vi "test4-SyncMessageWithError_API.vi"(8 "error in (no error)":errorcluster, 11 "TestCase in":refnum<class "testcase-CSMMessage.lvclass">) -> (0 "error out":errorcluster, 3 "TestCase out":refnum<class "testcase-CSMMessage.lvclass">)   [LabVIEW 2017, in "testcase-CSMMessage.lvclass"]
uses:
  testcase-CSMMessage.lvclass
  src/user.lib/_NEVSTOP/Communicable State Machine(CSM)/AdvanceAPI/CSM - Make String Arguments Safe.vi
  src/user.lib/_NEVSTOP/Communicable State Machine(CSM)/AdvanceAPI/CSM - Keywords.vi
  <vilib>/addons/_JKI Toolkits/VI Tester/TestCase.llb/TestCase.lvclass
  src/user.lib/_NEVSTOP/Communicable State Machine(CSM)/Communicable State Machine.lvlib
  C:/Program Files (x86)/National Instruments/LabVIEW 2017/vi.lib/addons/_JKI Toolkits/VI Tester/TestCase.llb/TestCase.lvclass
panel:
  out "LoopCount":i32
  out "Source CSM modules":string[](array[string])
  out "concatenated string":string
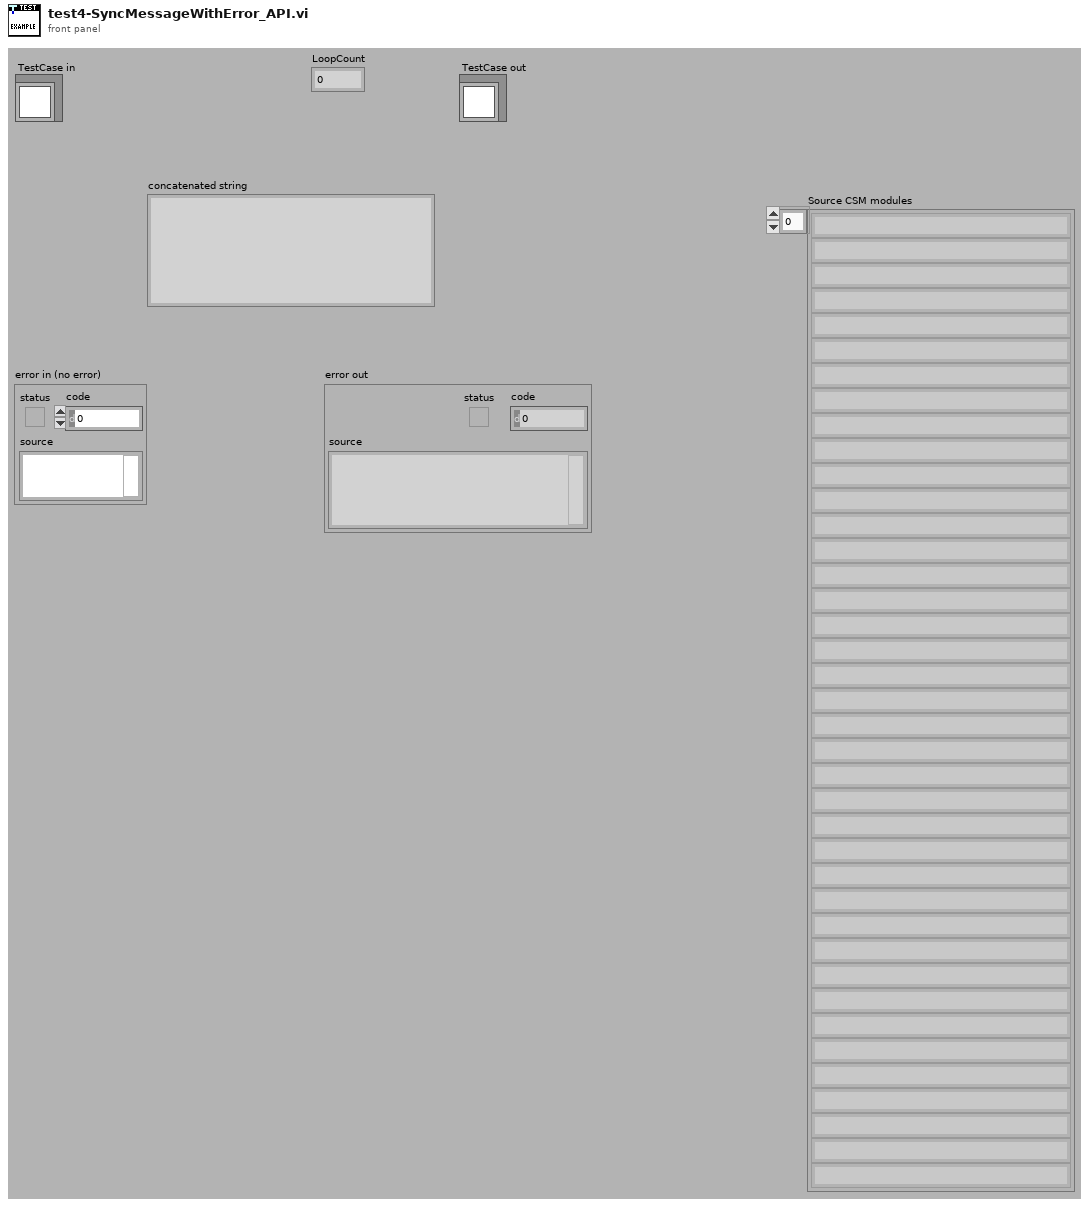
[diagram p1: front panel]
types:
  T1 = cluster{"Arguments":string, "Response":string, "error":errorcluster}
  T2 = cluster{"status":bool, "code":bool, "source":bool}
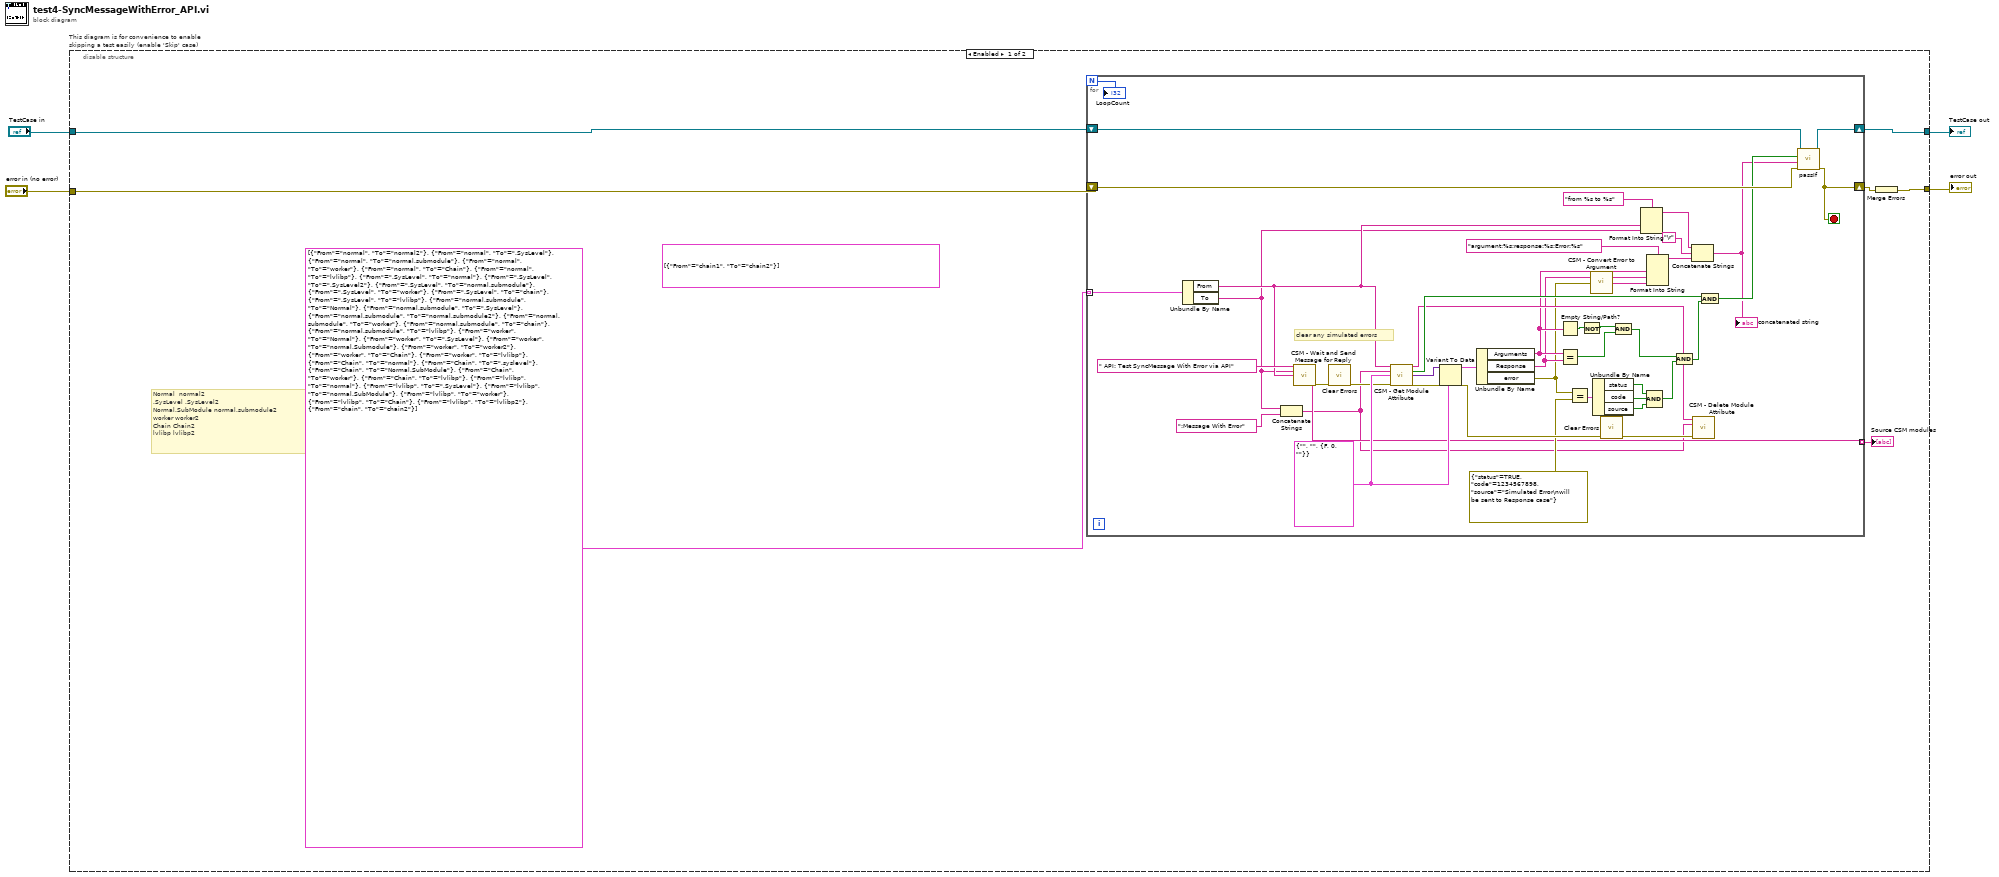
[diagram p0: block diagram]
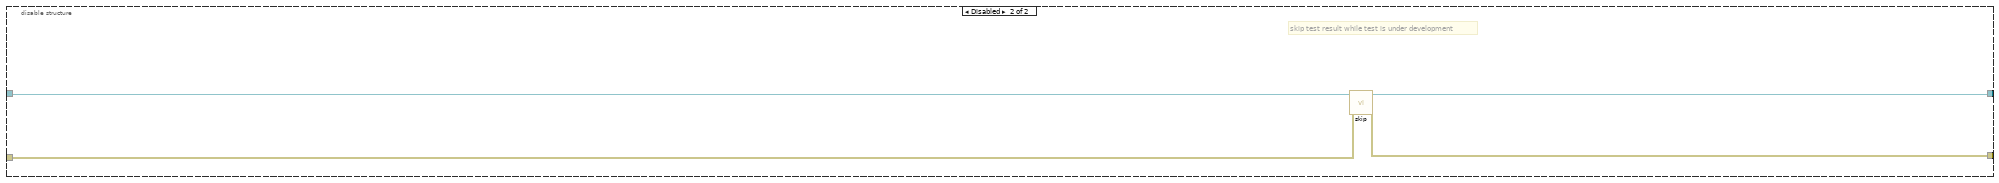
[diagram p2: hidden frame]
diagram:
  n1 = disable-structure "This diagram is for convenience to enable skipping a test easily (enable 'Skip' case)" shown="Enabled" {
    disable-tunnel: "TestCase in" -> [w11 w59]
    disable-tunnel: [w10 w57] -> w1
    disable-tunnel: [w7 w58] -> w3
    disable-tunnel: "error in (no error)" -> [w8 w56]
    frame Enabled {
      (unwired) cluster{"From":string, "To":string}[] [{"From"="chain1", "To"="chain2"}]
      # "Normal  normal2\n.SysLevel .SysLevel2\nNormal.SubModule normal.submodule2\nworker worker2\nChain Chain2\nlvlibp lvlibp2"
      n2 = for {
        N -> [w12]
        tunnel: cluster{"From":string, "To":string}[] [{"From"="normal", "To"="normal2"}, {"From"="normal", "To"=".SysLevel"}, {"From"="normal", "To"="normal.submodule"}, {"From"="normal", "To"="worker"}, {"From"="normal", "To"="Chain"}, {"From"="normal", "To"="lvlibp"}, {"From"=".SysLevel", "To"="normal"}, {"From"=".SysLevel", "To"=".SysLevel2"}, {"From"=".SysLevel", "To"="normal.submodule"}, {"From"=".SysLevel", "To"="worker"}, {"From"=".SysLevel", "To"="chain"}, {"From"=".SysLevel", "To"="lvlibp"}, {"From"="normal.submodule", "To"="Normal"}, {"From"="normal.submodule", "To"=".SysLevel"}, {"From"="normal.submodule", "To"="normal.submodule2"}, {"From"="normal.submodule", "To"="worker"}, {"From"="normal.submodule", "To"="chain"}, {"From"="normal.submodule", "To"="lvlibp"}, {"From"="worker", "To"="Normal"}, {"From"="worker", "To"=".SysLevel"}, {"From"="worker", "To"="normal.Submodule"}, {"From"="worker", "To"="worker2"}, {"From"="worker", "To"="Chain"}, {"From"="worker", "To"="lvlibp"}, {"From"="Chain", "To"="normal"}, {"From"="Chain", "To"=".syslevel"}, {"From"="Chain", "To"="Normal.SubModule"}, {"From"="Chain", "To"="worker"}, {"From"="Chain", "To"="lvlibp"}, {"From"="lvlibp", "To"="normal"}, {"From"="lvlibp", "To"=".SysLevel"}, {"From"="lvlibp", "To"="normal.SubModule"}, {"From"="lvlibp", "To"="worker"}, {"From"="lvlibp", "To"="Chain"}, {"From"="lvlibp", "To"="lvlibp2"}, {"From"="chain", "To"="chain2"}] -> [w44] mode=indexing
        shift-right: [w54] -> w10
        shift-left: w11 -> [w55]
        shift-right: [w27] -> w9
        shift-left: w8 -> [w53]
        tunnel: [w16] -> w6 mode=indexing
        stop <- w27 stop-if-true
        w50 = T1 {"Arguments"="", "Response"="", "error"={"status"=FALSE, "code"=0, "source"=""}}
        # "clear any simulated errors"
        n3 = Unbundle By Name(w44) -> ("From"=w17:string, "To"=w14:string)
        n4 = Concatenate Strings(w14, ":Message With Error" ("State")) -> (w13:string)
        n5 = call "CSM - Wait and Send Message for Reply.vi"("State"=" API: Test SyncMessage With Error via API", "Arguments (\"\")"=w14, "Target Module"=w17) -> (">> Source CSM >>"=w16:string, "error out"=w19:errorcluster)  [unwired: 10 in, 1 out]
        n6 = call <vilib>:"Clear Errors.vi"("error in (no error)"=w19) -> ("error out"=w18:errorcluster)  [unwired: 5 in, 1 out]
        n7 = call "CSM - Get Module Attribute.vi"("CSM Name"=w17, "Attribute"=w13, "Default Value (Empty Variant)"=w50, "Error In"=w18) -> ("CSM Name (Dup)"=w42:string, "Found"=w47:bool, "Value"=w49:variant, "error out"=w51:errorcluster)  [unwired: 7 in, 1 out]
        n8 = Variant To Data(error in=w51, type=w50, Variant=w49) -> (data=w48:T1, error out=w29:errorcluster)
        n9 = Unbundle By Name(w48) -> ("Arguments"=w37:string, "Response"=w36:string, "error"=w26:errorcluster)
        n10 = Empty String/Path?(string/path=w37) -> (empty?=w41:bool)
        n11 = Equal?(x=w37, y=w36) -> (x = y?=w39:bool)
        n12 = Equal?(x=w26, y=errorcluster {"status"=TRUE, "code"=1234567898, "source"="Simulated Error\nwill be sent to Response case"} ("error out")) -> (x = y?=w24:T2)
        n13 = Not(x=w41) -> (.not. x?=w40:bool)
        n14 = call "CSM - Convert Error to Argument.vi"("Error"=w26) -> ("Argument"=w35:string)  [unwired: 4 in]
        n15 = Unbundle By Name(w24) -> ("status"=w23:bool, "code"=w22:bool, "source"=w21:bool)
        n16 = call <vilib>:"Clear Errors.vi"("error in (no error)"=w29) -> ("error out"=w28:errorcluster)  [unwired: 5 in, 1 out]
        n17 = And(x=w40, y=w39) -> (x .and. y?=w38:bool)
        n18 = Format Into String(format string="from %s to %s", w17, w14) -> (resulting string=w31:string)  [unwired: 2 in, 1 out]
        n19 = Format Into String(format string="argument:%s;response:%s;Error:%s", w37, w36, w35) -> (resulting string=w34:string)  [unwired: 2 in, 1 out]
        n20 = Compound Arithmetic op=AND(w23, w22, w21) -> (w20:bool)
        n21 = And(x=w38, y=w20) -> (x .and. y?=w46:bool)
        n22 = Concatenate Strings(w31, "\r", w34) -> (w32:string)
        "concatenated string" <- w32
        n23 = call "CSM - Delete Module Attribute.vi"("CSM Name"=w42, "Attribute"=w13, "Error In"=w28) -> ()  [unwired: 9 in, 4 out]
        n24 = And(x=w47, y=w46) -> (x .and. y?=w45:bool)
        n25 = call-dynamic "passIf.vi"("error in (no error)"=w53, "message (\"\")"=w32, "pass"=w45, "TestCase in"=w55) -> ("error out"=w27:errorcluster, "TestCase out"=w54:refnum<class "testcase-CSMMessage.lvclass">)  [unwired: 6 in]
        "LoopCount" <- w12
      }
      "Source CSM modules" <- w6
      n26 = Merge Errors(w9) -> (w7:errorcluster)
    }
    frame Disabled {
      # "skip test result while test is under development"
      n27 = call <vilib>:"skip.vi"("error in (no error)"=w56, "TestCase in"=w59) -> ("error out"=w58:errorcluster, "TestCase out"=w57:refnum<class "testcase-CSMMessage.lvclass">)  [unwired: 8 in]
    }
  }
  "error out" <- w3
  "TestCase out" <- w1
